vi "test_RFID.vi"() -> ()   [LabVIEW 2015]
uses:
  Library/IF2_Reader/IF2_Reader.lvlib
panel:
  out "TagData out":cluster{"TagCode":string, "FirstSeemUs":u64}[](array[cluster])
  out "connection ID":refnum<k5>
  out "OK Button 2":bool
  in  "OK Button":bool
  out "parar":bool
  out "TagArray":string[](array[string])
  in  "stop":bool
  in  "IP RFID":string="172.23.3.203"
  in  "Puerto RFID":u16=2189
  out "Report":string
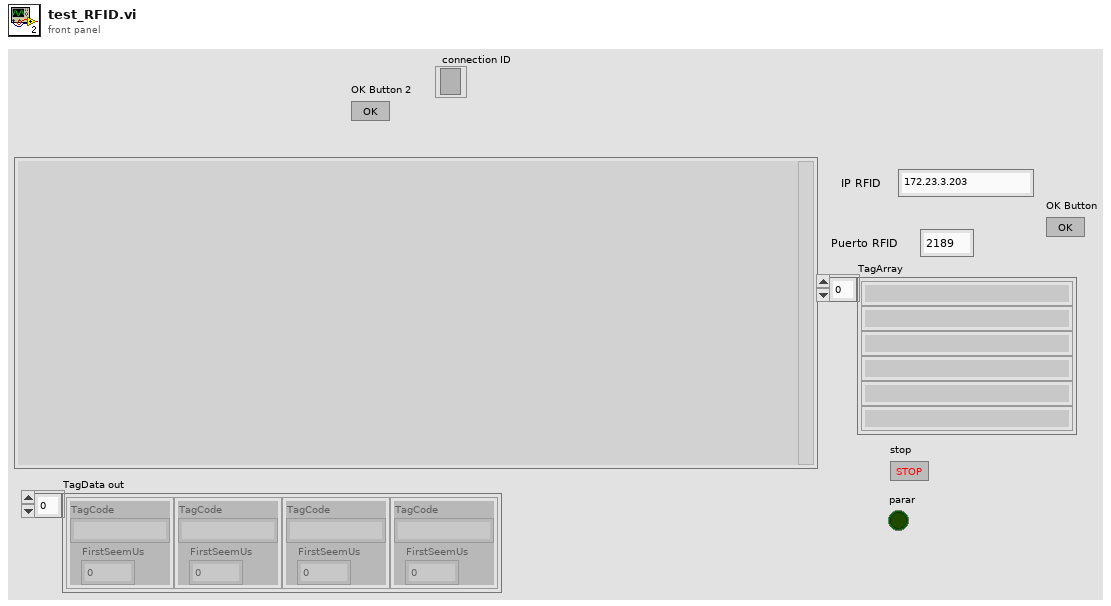
[diagram p1: front panel]
types:
  T1 = cluster{"IP":string, "Port":u16, "ReaderConfigFile":path, "ROspecConfigFile":path}
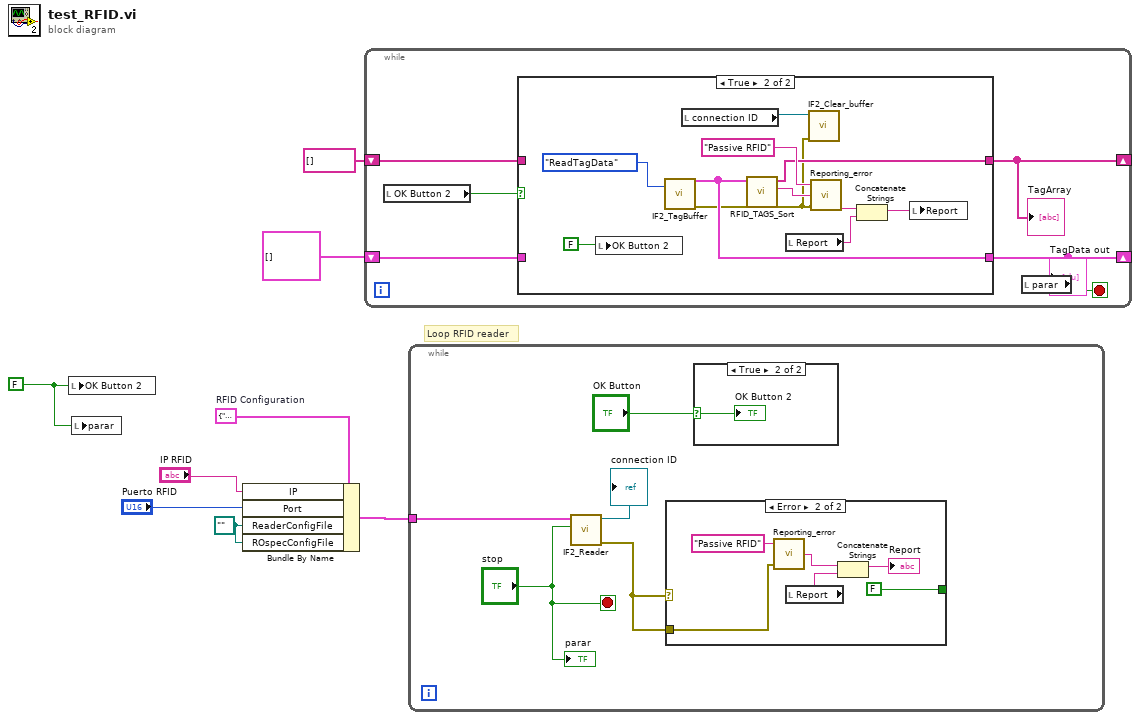
[diagram p0: block diagram]
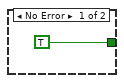
[diagram p4: hidden frame]
diagram:
  w3 = FALSE ("Boolean")
  w8 = T1 {"IP"="169.254.1.1", "Port"=5084, "ReaderConfigFile"=path "", "ROspecConfigFile"=path ""}  # RFID Configuration
  w6 = path "" ("ReaderConfigFile")
  # "Loop RFID reader"
  n1 = local write "OK Button 2"(w3) -> ()
  n2 = local write "parar"(w3) -> ()
  n3 = Bundle By Name(cluster=w8, "IP"="IP RFID", "Port"="Puerto RFID", "ReaderConfigFile"=w6, "ROspecConfigFile"=w6) -> (w7:T1)
  n4 = while {
    shift-right: [w12] -> _
    shift-left: string[] [] ("TagArray") -> [w11]
    shift-right: [w10] -> _
    shift-left: cluster{"TagCode":string, "FirstSeemUs":u64}[] [] ("TagData out") -> [w9]
    stop <- w14 stop-if-true
    n5 = local read "OK Button 2"() -> (w13:bool)
    n6 = case shown="True" w13 {
      tunnel: [w16 w21] -> w12
      tunnel: [w15 w20] -> w10
      tunnel: w11 -> [w16 _]
      tunnel: w9 -> [w15 _]
      frame False {
      }
      frame True {
        n7 = local write "OK Button 2"(FALSE ("Boolean")) -> ()
        n8 = call "IF2_TagBuffer.vi"("Action"=enum16{"Init", "WriteTagData", "ReadTagData"}."ReadTagData") -> ("error out"=w18:errorcluster, "TagData out"=w20:cluster{"TagCode":string, "FirstSeemUs":u64}[])  [unwired: 9 in]
        n9 = local read "connection ID"() -> (w17:refnum<k5>)
        n10 = call "RFID_TAGS_Sort.vi"("TagData in"=w20) -> ("TagString"=w22:string, "TagArray"=w21:string[])  [unwired: 9 in]
        n11 = local read "Report"() -> (w23:string)
        n12 = call "IF2_Clear_buffer.vi"("error in (no error)"=w18, "TCP Network Connection in"=w17) -> ()  [unwired: 8 in, 2 out]
        n13 = call "Reporting_error.vi"("error out 2"=w18, "Concept explanation"=w22, "Concept"="Passive RFID") -> ("Reporting"=w26:string)
        n14 = Concatenate Strings(w26, w23) -> (w24:string)
        n15 = local write "Report"(w24) -> ()
      }
    }
    "TagArray" <- w12
    "TagData out" <- w10
    n16 = local read "parar"() -> (w14:bool)
  }
  n17 = while {
    tunnel: w7 -> [w31]
    stop <- "stop" stop-if-true
    n18 = call "IF2_Reader.vi"("Stop"="stop", "RFID Configuration"=w31) -> ("error out"=w32:errorcluster, "connection ID"=→"connection ID":refnum<k5>)  [unwired: 8 in]
    n19 = case shown="Error" w32 {
      tunnel: w32 -> [_ w36]
      tunnel: [TRUE ("RFIDStatus") FALSE ("RFIDStatus")] -> _
      frame No Error {
      }
      frame Error {
        n20 = call "Reporting_error.vi"("error out 2"=w36, "Concept"="Passive RFID") -> ("Reporting"=w37:string)  [unwired: 1 in]
        n21 = local read "Report"() -> (w38:string)
        n22 = Concatenate Strings(w37, w38) -> (→"Report":string)
      }
    }
    n23 = case shown="True" "OK Button" {
      selector: "OK Button" -> [_ w33]
      frame False {
      }
      frame True {
        "OK Button 2" <- w33
      }
    }
    "parar" <- "stop"
  }
